vi "Multiple_File_Opener.vi"() -> ()   [LabVIEW 2023]
uses:
  <vilib>/Utility/file.llb/Read Delimited Spreadsheet (string).vi
panel:
  in  "Base Folder":path=path "C:/Users/AIIH/Documents/LabVIEW/EEG/Filtered_Data"
  out "appended path":path
  in  "Boolean":bool
  in  "Files":path=path "C:/Users/AIIH/Documents/LabVIEW/EEG/RECORDS_1.csv"
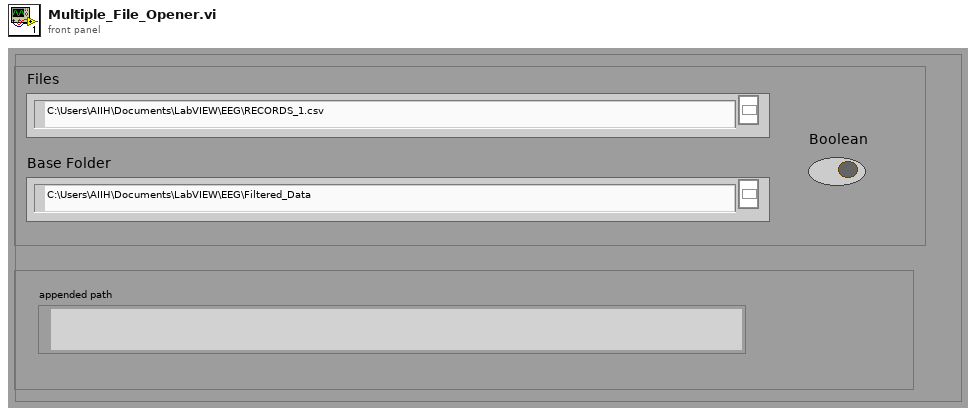
[diagram p1: front panel]
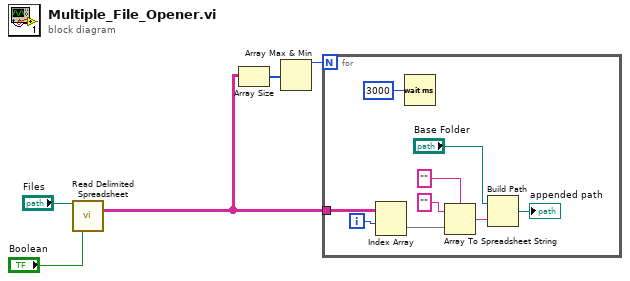
[diagram p0: block diagram]
diagram:
  n1 = call-poly <vilib>:"Read Delimited Spreadsheet.vi"("file path (dialog if empty)"="Files", "transpose? (F)"="Boolean") -> ("all rows"=w3:string[][])  [unwired: 8 in, 5 out]
  n2 = Array Size(array=w3) -> (size(s)=w2:i32[])
  n3 = Array Max & Min(array=w2) -> (max value=w1:i32)  [unwired: 3 out]
  n4 = for {
    N: w1 -> [_]
    tunnel: w3 -> [w14]
    i -> [w13]
    n5 = Index Array(array=w14, index (row)=w13) -> (element=w10:string[])  [unwired: 1 in]
    n6 = Wait (ms)(milliseconds to wait=u32 3000) -> ()  [unwired: 1 out]
    n7 = Array To Spreadsheet String(delimiter (Tab)="", array=w10, 3:"" ("format string")) -> (spreadsheet string=w11:string)
    n8 = Build Path(base path="Base Folder", name or relative path=w11) -> (appended path=→"appended path":path)
  }
